vi "HexToString.vi"(10 "字符个数":i32=6, 11 "数组":u16[](array[numeric]) format="%04xH") -> (3 "STRING":string[](array[string]))   [LabVIEW 2016, in "斯坦道总磷.lvlib"]
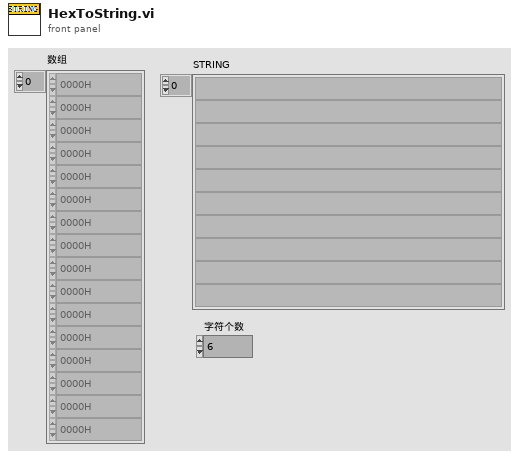
[diagram p1: front panel]
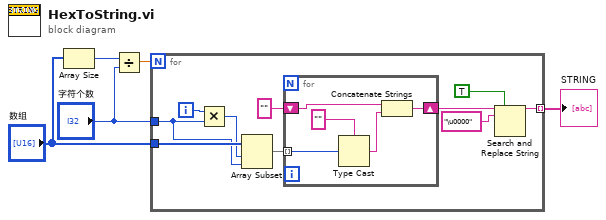
[diagram p0: block diagram]
diagram:
  n1 = Array Size(array="数组") -> (size(s)=w5:i32)
  n2 = Divide(x=w5, y="字符个数") -> (x/y=w4:dbl)
  n3 = for {
    N: w4 -> [_]
    tunnel: "数组" -> [w15]
    tunnel: [w9] -> w3 mode=indexing
    tunnel: "字符个数" -> [w6]
    i -> [w14]
    n4 = Multiply(x=w14, y=w6) -> (x*y=w13:i32)
    n5 = Array Subset(array=w15, index=w13, length=w6) -> (w11:u16[])
    n6 = for {
      shift-right: [w20] -> w10
      shift-left: "" -> [w17]
      tunnel: w11 -> [w19] mode=indexing
      n7 = Type Cast(type="", x=w19) -> (*(type *) &x=w16:string)
      n8 = Concatenate Strings(w17, w16) -> (w20:string)
    }
    n9 = Search and Replace String(replace all?=TRUE ("替换全部？(F)"), input string=w10, search string="\u0000" ("搜索字符串")) -> (result string=w9:string)  [unwired: 5 in, 3 out]
  }
  "STRING" <- w3
